vi "importESDU.vi"(1 "ESDU Path":path=path "" caption="start path") -> (0 "ESDU Mean Factors":string[][](array[string]))   [LabVIEW 2018]
uses:
  <vilib>/addons/_office/excel.llb/Excel Get Data ([str]).vi
  <vilib>/Utility/NIReport.llb/NI_report.lvclass
  <vilib>/Utility/NIReport.llb/Excel/NI_Excel.lvclass
  <vilib>/addons/_office/NI_ReportGenerationToolkit.lvlib
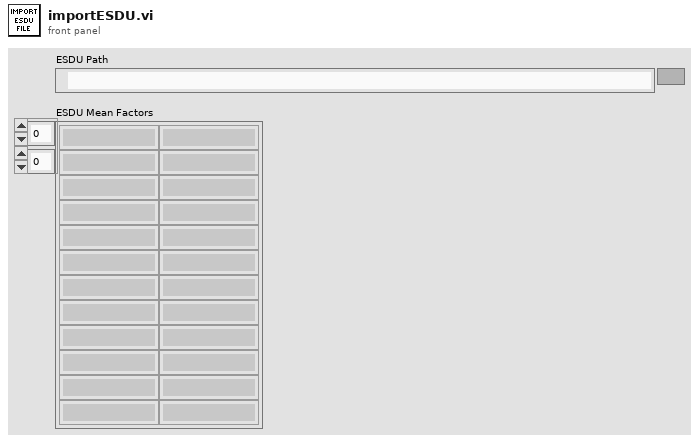
[diagram p1: front panel]
types:
  T1 = enum16{"Standard Report", "HTML", "Word", "Excel"}
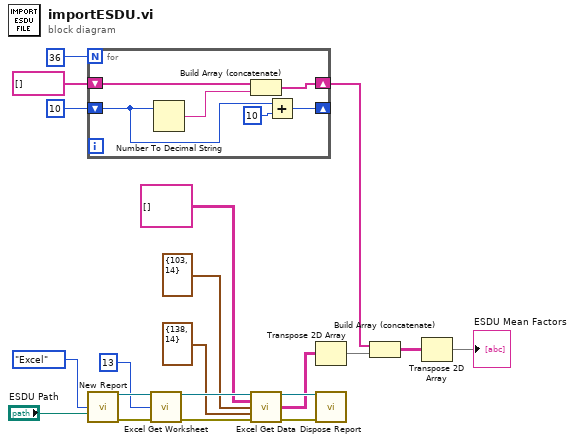
[diagram p0: block diagram]
diagram:
  n1 = for {
    N: 36 -> [_]
    shift-right: [w25] -> _
    shift-left: 10 -> [w23]
    shift-right: [w22] -> w6
    shift-left: string[] [] -> [w21]
    n2 = Number To Decimal String(number=w23) -> (decimal integer string=w24:string)  [unwired: 1 in]
    n3 = Build Array (concatenate)(w21, w24) -> (w22:string[])
    n4 = Add(x=w23, y=10) -> (x+y=w25:i32)
  }
  n5 = call <vilib>:"New Report.vi"("report type"=T1."Excel", "template (empty)"="ESDU Path") -> ("report out"=w15:refnum<class "NI_report.lvclass">, "error out"=w17:errorcluster)  [unwired: 4 in, 8 out]
  n6 = call <vilib>:"Excel Get Worksheet.vi"("report in"=w15, "worksheet index (0)"=13, "error in (no error)"=w17) -> ("report out"=w16:refnum<class "NI_report.lvclass">, "error out"=w18:errorcluster)  [unwired: 11 out]
  n7 = call-poly <vilib>:"Excel Get Data.vi"("report in"=w16, "data type"=string[][] [], "start (-1, -1)"=cluster{"row":i32, "column":i32} {"row"=103, "column"=14}, "end (-1, -1)"=cluster{"row":i32, "column":i32} {"row"=138, "column"=14}, "error in (no error)"=w18) -> ("report out"=w19:refnum<class "NI_report.lvclass">, "data"=w5:string[][], "error out"=w20:errorcluster)  [unwired: 8 out]
  n8 = Transpose 2D Array(2D array=w5) -> (transposed array=w4:string[][])
  n9 = call-dynamic "Dispose Report.vi"("report in"=w19, "error in (no error)"=w20) -> ()  [unwired: 3 in, 11 out]
  n10 = Build Array (concatenate)(w6, w4) -> (w3:string[][])
  n11 = Transpose 2D Array(2D array=w3) -> (transposed array=→"ESDU Mean Factors":string[][])
